vi "Main On Compile Action VI.vi"(8 "error in (no error)":errorcluster, 11 "Device Item Ref in":T1 format="%.0x") -> (0 "error out":errorcluster, 3 "Item Ref out":T1=18446744073709551615 format="%.0x")   [LabVIEW 2010, in "Sensor Simulation Custom Device.lvlib"]
uses:
  Sensor Simulation Custom Device.lvlib
  <vilib>/NI Veristand/Custom Device API/Custom Device Item Ref.ctl
  <vilib>/NI Veristand/Custom Device API/Custom Device API.lvlib
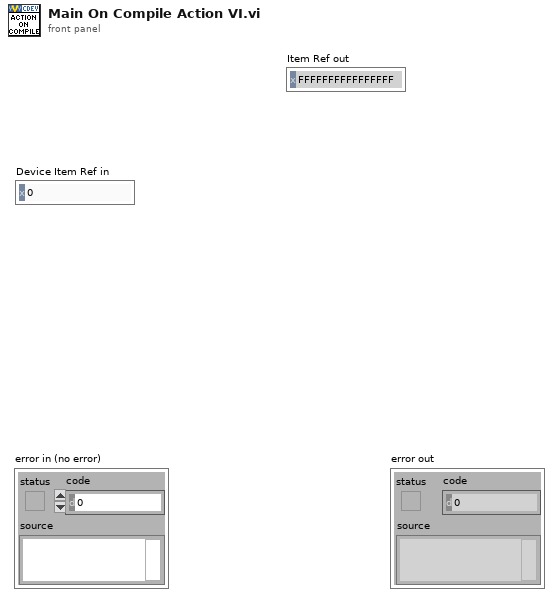
[diagram p1: front panel]
types:
  T1 = typedef "Custom Device API.lvlib/Custom Device Item Ref.ctl" = u64
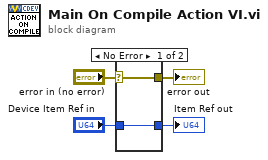
[diagram p0: block diagram]
diagram:
  n1 = case shown="No Error" "error in (no error)" {
    selector: "error in (no error)" -> [w5 w8]
    tunnel: [w5 w8] -> w3
    tunnel: "Device Item Ref in" -> [w6 w7]
    tunnel: [w6 w7] -> w1
    frame No Error {
    }
    frame Error {
    }
  }
  "error out" <- w3
  "Item Ref out" <- w1
